vi "Hardware Types Request.vi"(8 "error in (no error)":errorcluster, 9 "Requested Types":string[](array[string]), 10 "Requestor":string, 11 "Mag Lab Measure Controller in":refnum<class "Mag Lab Measure Controller.lvclass">) -> (0 "error out":errorcluster, 3 "Mag Lab Measure Controller out":refnum<class "Mag Lab Measure Controller.lvclass">)   [LabVIEW 2015, in "Mag Lab Measure Controller.lvclass"]
uses:
  Mag Lab Measure Controller.lvclass
  Mag Lab Measurement Messages/Matching Hardware Callback Msg/Matching Hardware Callback Msg.lvclass/Matching Hardware Callback Msg.ctl
  <vilib>/ActorFramework/Message Enqueuer/Message Enqueuer.lvclass/Message Enqueuer.ctl
  <vilib>/ActorFramework/Message Enqueuer/Enqueue.vi
  <vilib>/ActorFramework/Message Priority Queue/Priority Enqueue.vi
  Mag Lab Measurement Messages/Matching Hardware Callback Msg/Matching Hardware Callback Msg.lvclass
  Mag Lab Measure Base/Mag Lab Measure Base.lvclass
  Mag Lab Error Handler/Mag Lab Error Handler.lvclass
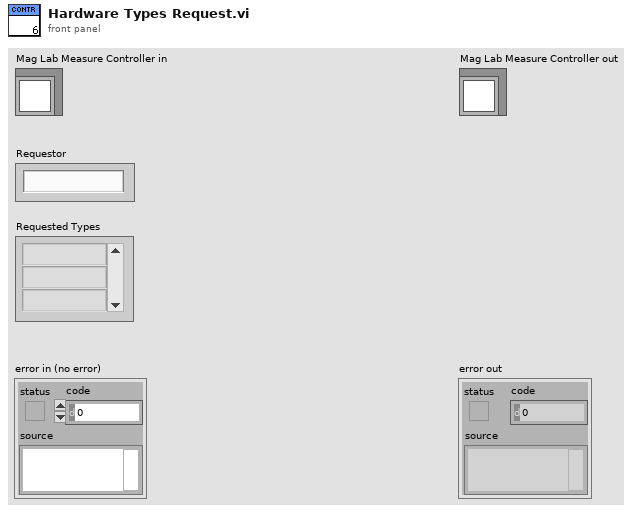
[diagram p1: front panel]
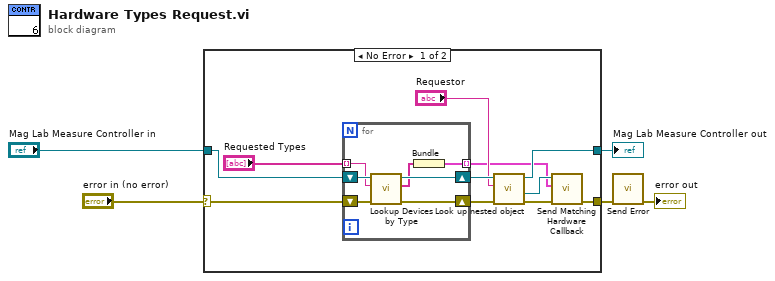
[diagram p0: block diagram]
diagram:
  n1 = case shown="No Error" "error in (no error)" {
    selector: "error in (no error)" -> [w14 w25]
    tunnel: [w6 w25] -> w2
    tunnel: [w10 w24] -> w3
    tunnel: "Mag Lab Measure Controller in" -> [w16 w24]
    frame No Error {
      n2 = for {
        shift-right: [w22] -> w13
        shift-left: w16 -> [w23]
        tunnel: "Requested Types" -> [w21] mode=indexing
        tunnel: [w19] -> w8 mode=indexing
        shift-right: [w17] -> w11
        shift-left: w14 -> [w18]
        n3 = call "Lookup Devices by Type.vi"("error in (no error)"=w18, "Hardware Type"=w21, "Mag Lab Measure Controller in"=w23) -> ("error out"=w17:errorcluster, "Matching Devices"=w20:string[], "Mag Lab Measure Controller out"=w22:refnum<class "Mag Lab Measure Controller.lvclass">)  [unwired: 6 in]
        n4 = Bundle("Matching Devices"=w20) -> (w19:cluster{"Matching Devices":string[]})  [unwired: 1 in]
      }
      n5 = call "Look up nested object.vi"("error in (no error)"=w11, "Object name"="Requestor", "Mag Lab Measure Base in"=w13) -> ("error out"=w7:errorcluster, "Object Queue"=w9:refnum<class "Message Enqueuer.lvclass">, "Mag Lab Measure Base out"=w10:refnum<class "Mag Lab Measure Controller.lvclass">)  [unwired: 5 in, 1 out]
      n6 = call "Send Matching Hardware Callback.vi"("error in (no error)"=w7, "Match"=w8, "Message Enqueuer"=w9) -> ("error out"=w6:errorcluster)  [unwired: 7 in, 1 out]
    }
    frame Error {
    }
  }
  "Mag Lab Measure Controller out" <- w3
  n7 = call "Send Error.vi"("error in (no error)"=w2) -> ("error out"=→"error out":errorcluster)  [unwired: 9 in, 1 out]
